vi "Pause.vi"() -> ()   [LabVIEW 2017]
panel:
  out "millisecond timer value":u32
  out "Sweep No":i32
  in  "stop":bool
  in  "Seconds to Wait":i32=1000
  out "Seconds":i32
  out "Minutes":i32
  out "Hours":i32
  in  "Delay (ms)":u32=5000
  in  "Pause/Continue":bool
  out "Time Stamp":timestamp format="%<%.3X>T"
  out "output array":string[][](array[string])
  in  "Number of Sweeps":i32=1 min=1 max=1000 step=1
  in  "Number of Points":i32=50 min=10 max=10000 step=1
  out "Graph":cluster{"Y":dbl[], "Y":dbl[]}[](graph)
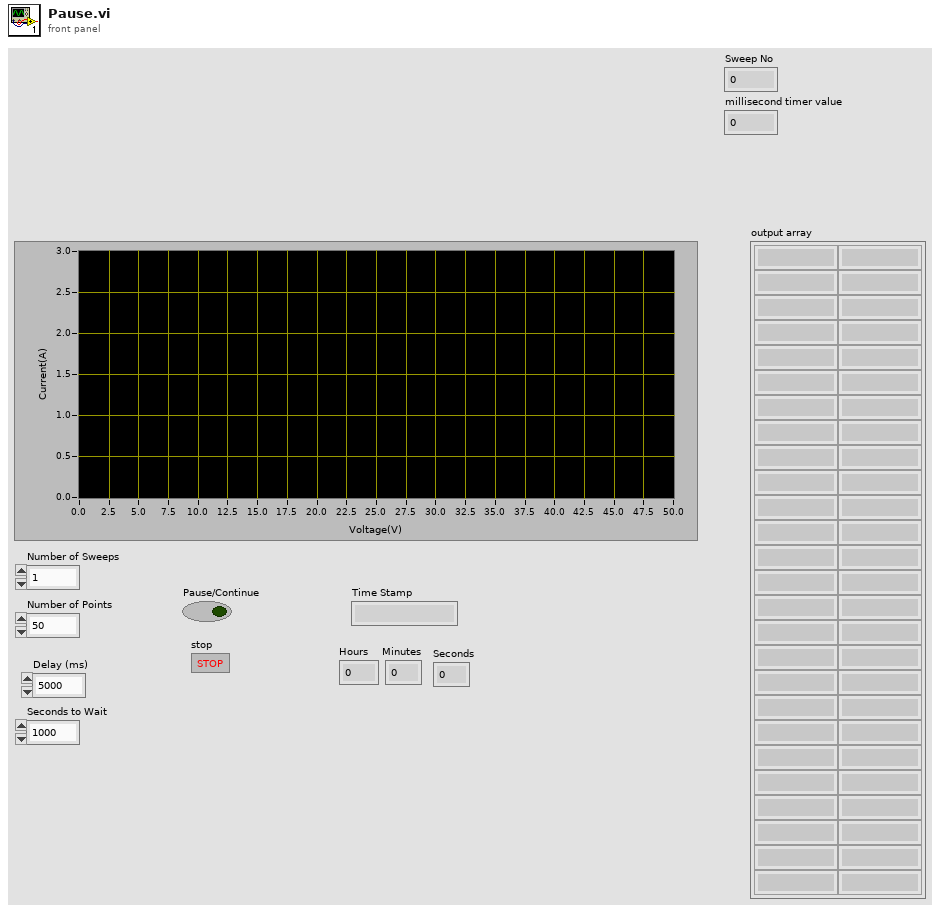
[diagram p1: front panel]
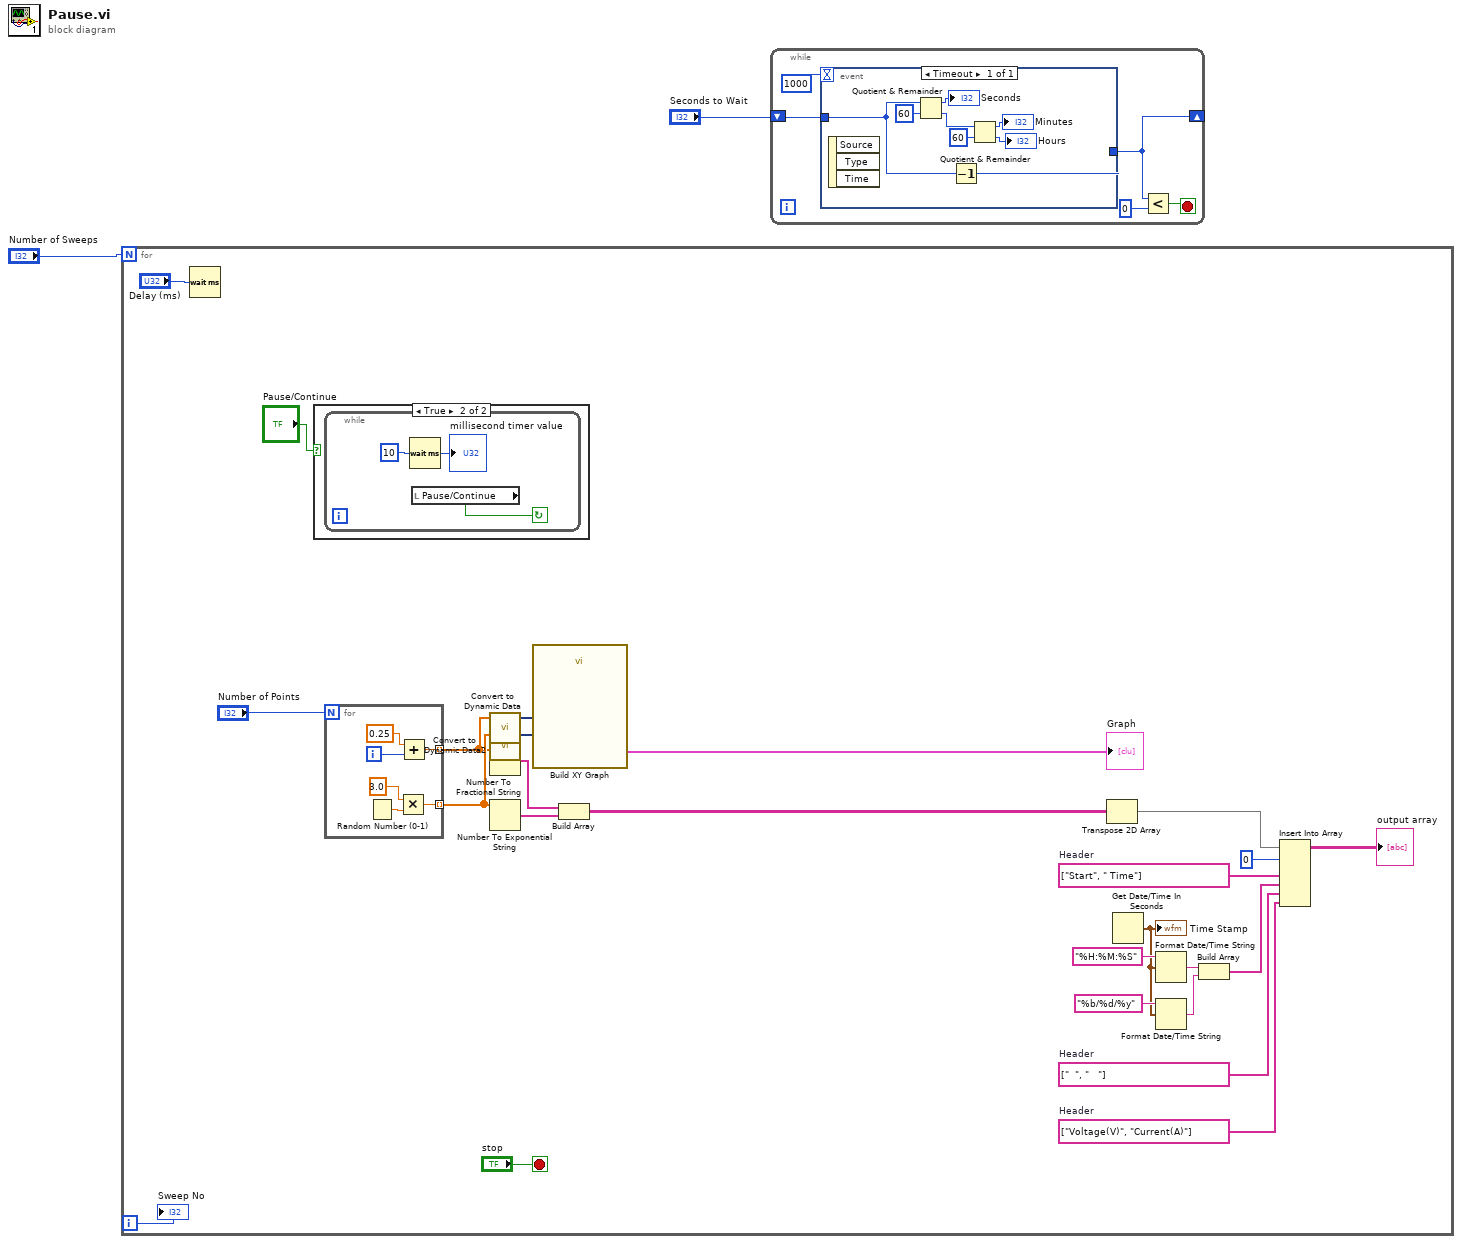
[diagram p0: block diagram]
diagram:
  n1 = for {
    N: "Number of Sweeps" -> [_]
    i -> [w3]
    stop <- "stop" stop-if-true
    w10 = string[] ["  ", "   "]  # Header
    w12 = string[] ["Start", " Time"]  # Header
    w9 = string[] ["Voltage(V)", "Current(A)"]  # Header
    n2 = Wait (ms)(milliseconds to wait="Delay (ms)") -> ()  [unwired: 1 out]
    n3 = case shown="True" "Pause/Continue" {
      frame False {
      }
      frame True {
        n4 = while {
          stop <- w30 continue-if-true
          n5 = Wait (ms)(milliseconds to wait=u32 10) -> (millisecond timer value=→"millisecond timer value":u32)
          n6 = local read "Pause/Continue"() -> (w30:bool)
        }
      }
    }
    n7 = for {
      N: "Number of Points" -> [_]
      tunnel: [w32] -> w7 mode=indexing
      tunnel: [w31] -> w20 mode=indexing
      i -> [w33]
      n8 = Random Number (0-1)() -> (number: 0 to 1=w34:dbl)
      n9 = Multiply(x=3.0, y=w34) -> (x*y=w31:dbl)
      n10 = Add(x=0.25 ("y"), y=w33) -> (x+y=w32:dbl)
    }
    n11 = call "Convert to Dynamic Data"("Array"=w7) -> ("Dynamic Data Type"=w27:dynamicdata)  [unwired: 3 in]
    n12 = call "Convert to Dynamic Data2"("Array"=w20) -> ("Dynamic Data Type"=w26:dynamicdata)  [unwired: 3 in]
    n13 = Number To Fractional String(number=w7) -> (F-format string=w19:string[])  [unwired: 3 in]
    n14 = Number To Exponential String(number=w20) -> (E-format string=w18:string[])  [unwired: 3 in]
    n15 = call "Build XY Graph"("Y Input"=w26, "X Input"=w27) -> ("XY Graph"=→"Graph":cluster{"X":dbl[], "Y":dbl[]}[])  [unwired: 8 in, 1 out]
    n16 = Build Array(w19, w18) -> (w22:string[][])
    n17 = Transpose 2D Array(2D array=w22) -> (transposed array=w23:string[][])
    n18 = Get Date/Time In Seconds() -> (seconds since 1Jan1904=w13:timestamp)
    "Time Stamp" <- w13
    n19 = Format Date/Time String(time format string (%c)="%H:%M:%S", seconds (now)=w13) -> (date/time string=w16:string)  [unwired: 1 out]
    n20 = Format Date/Time String(time format string (%c)="%b/%d/%y", seconds (now)=w13) -> (date/time string=w15:string)  [unwired: 1 out]
    n21 = Build Array(w16, w15) -> (w11:string[])
    n22 = Insert Into Array "Insert Into Array"(array=w23, index (row)=0, new element #1=w12, new element #2=w11, new element #3=w10, new element #4=w9) -> (→"output array":string[][])  [unwired: 1 in]
    "Sweep No" <- w3
  }
  n23 = while {
    shift-right: [w38] -> _
    shift-left: "Seconds to Wait" -> [w40]
    stop <- w39 stop-if-true
    n24 = event shown="[0] Timeout" {
      selector: _ -> [_]
      dyn-events: _ -> [_]
      timeout: 1000 -> [_]
      tunnel: w40 -> [w47]
      tunnel: [w49] -> w38
      event Timeout {
        n25 = event-data() -> ()  [unwired: 1 in, 3 out]
        n26 = Quotient & Remainder(x=w47, y=60) -> (x-y*floor(x/y)=→"Seconds":i32, floor(x/y)=w43:i32)
        n27 = Decrement(x=w47) -> (x-1=w49:i32)
        n28 = Quotient & Remainder(x=w43, y=60) -> (x-y*floor(x/y)=→"Minutes":i32, floor(x/y)=→"Hours":i32)
      }
    }
    n29 = Less?(x=w38, y=0) -> (x < y?=w39:bool)
  }
